vi "WLAN_FrameBuild_SNR.vi"(8 "error in (no error)":errorcluster, 10 "Modulation parameter":T1, 11 "data in":i8[](array[numeric]) caption="input bit stream") -> (0 "error out":errorcluster, 2 "OFDM":cdb[](array[numeric]))   [LabVIEW 2018]
panel:
  out "size(s) 3":i32
  out "size(s) 2":i32
  out "size(s)":i32
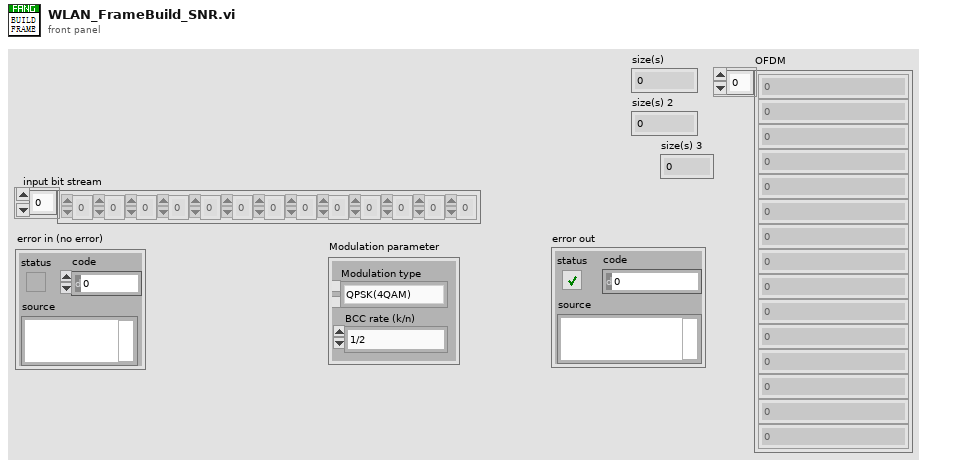
[diagram p1: front panel]
types:
  T1 = cluster{"Modulation type":enum16{"QPSK(4QAM)", "64QAM", "16QAM", "BPSK"}, "BCC rate (k/n)":enum16{"1/2", "2/3", "3/4"}}
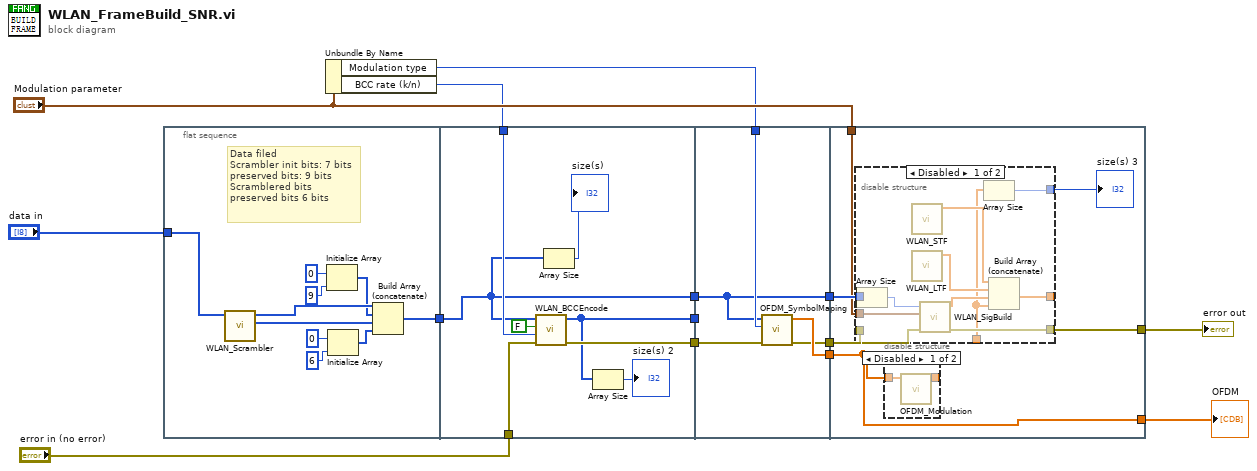
[diagram p0: block diagram]
diagram:
  n1 = flat-sequence {
    tunnel: "data in" -> [w24]
    tunnel: [w23] -> w13
    tunnel: w13 -> [w28]
    tunnel: "error in (no error)" -> [w31]
    tunnel: [w30] -> w11
    tunnel: [w26] -> w10
    tunnel: w7 -> [w29]
    tunnel: [w28] -> w3
    tunnel: w11 -> [w36]
    tunnel: w10 -> [_]
    tunnel: w8 -> [w37]
    tunnel: [w35] -> w6
    tunnel: [w34] -> w5
    tunnel: w3 -> [w33]
    tunnel: [w33] -> w2
    tunnel: "Modulation parameter" -> [w42]
    tunnel: w6 -> [w38]
    tunnel: w5 -> [w41]
    tunnel: [w40] -> w4
    tunnel: w2 -> [w43]
    tunnel: [w38] -> w1
    frame #0 {
      # "Data filed\nScrambler init bits: 7 bits\npreserved bits: 9 bits\nScramblered bits\npreserved bits 6 bits"
      n2 = call "WLAN_Scrambler.vi"("input bit stream"=w24) -> ("scrambled bits"=w18:i8[], "scrambler initial bit"=w22:i8[])  [unwired: 9 in]
      n3 = Initialize Array(i8 0 ("element"), 9 ("dimension size")) -> (w21:i8[])
      n4 = Initialize Array(i8 0 ("element"), 6 ("dimension size")) -> (w15:i8[])
      n5 = Build Array (concatenate)(w22, w21, w18, w15) -> (w23:i8[])
    }
    frame #1 {
      n6 = call "WLAN_BCCEncode.vi"("error in (no error)"=w31, "BCC rate (k/n)"=w29, "need add zeros?"=FALSE, "input bit stream"=w28) -> ("error out"=w30:errorcluster, "output bit stream 3"=w26:i8[])  [unwired: 6 in]
      n7 = Array Size(array=w28) -> (size(s)=→"size(s)":i32)
      n8 = Array Size(array=w26) -> (size(s)=→"size(s) 2":i32)
    }
    frame #2 {
      n9 = call "OFDM_SymbolMaping.vi"("error in (no error)"=w36, "Modulation type"=w37, "input bit stream"=w33) -> ("error out"=w34:errorcluster, "symbols"=w35:cdb[])  [unwired: 7 in]
    }
    frame #3 {
      n10 = disable-structure shown="Disabled" {
        disable-tunnel: w43 -> [w56 _]
        disable-tunnel: w42 -> [w54 _]
        disable-tunnel: w41 -> [w51 _]
        disable-tunnel: [w50 _] -> w40
        disable-tunnel: [w48 _] -> w39
        disable-tunnel: [w47 _] -> _
        disable-tunnel: _ -> [w46 _]
        frame Disabled {
          n11 = Array Size(array=w56) -> (size(s)=w55:i32)
          n12 = call "WLAN_STF.vi"() -> ("STF"=w52:cdb[])  [unwired: 11 in]
          n13 = call "WLAN_LTF.vi"() -> ("LTF"=w53:cdb[])  [unwired: 11 in]
          n14 = call "WLAN_SigBuild.vi"("Data bit length"=w55, "Modulation parameter"=w54, "error in (no error)"=w51) -> ("symbols"=w49:cdb[], "error out"=w50:errorcluster)  [unwired: 6 in]
          n15 = Array Size(array=w46) -> (size(s)=w48:i32)
          n16 = Build Array (concatenate)(w52, w53, w49, w46) -> (w47:cdb[])
        }
        frame Enabled {
        }
      }
      "size(s) 3" <- w39
      n17 = disable-structure shown="Disabled" {
        disable-tunnel: w38 -> [w45 _]
        disable-tunnel: [w44 _] -> _
        frame Disabled {
          n18 = call "OFDM_Modulation.vi"("Input sequence"=w45) -> ("Output sequence"=w44:cdb[])  [unwired: 10 in]
        }
        frame Enabled {
        }
      }
    }
  }
  n19 = Unbundle By Name("Modulation parameter") -> ("Modulation type"=w8:enum16{"QPSK(4QAM)", "64QAM", "16QAM", "BPSK"}, "BCC rate (k/n)"=w7:enum16{"1/2", "2/3", "3/4"})
  "error out" <- w4
  "OFDM" <- w1
